vi "proc.util.compare.vi"(8 "error in":errorcluster, 9 "stepElement in":variant, 10 "Input":dbl, 11 "procElement in":variant) -> (0 "error out":errorcluster, 1 "stepElement out":variant, 2 "resulting string":string, 3 "procElement out":variant, 4 "Next State":cluster{"CMD":T1, "data":variant})   [LabVIEW 2024]
uses:
  controls/typeCmdPostStepFunc.ctl
  controls/typeStepVarients.ctl
  Polymorphics/variantCtrlString.vi
  proc.util.validateParamExist.vi
  <vilib>/Utility/error.llb/Clear Errors.vi
  util.error.create.vi
  controls/typeProcVarientName.ctl
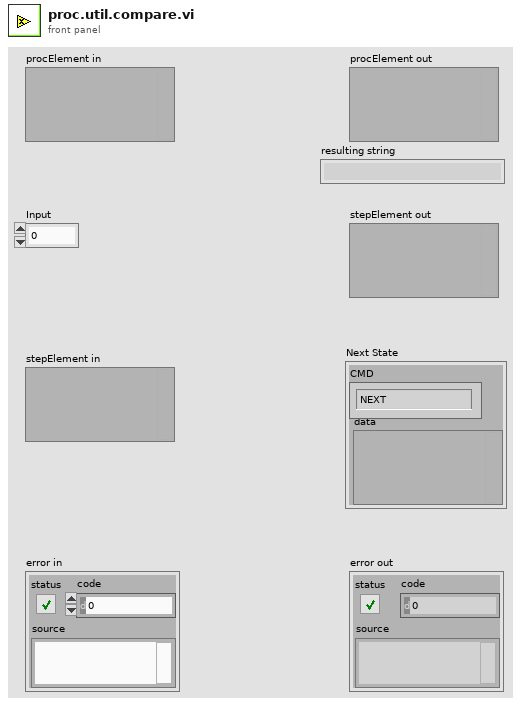
[diagram p1: front panel]
types:
  T1 = typedef "typeCmdPostStepFunc.ctl" = enum16{"NEXT", "PREV", "JUMP", "STAY", "COMPLETE", "ENGCALL.PROC.START", "ENGCALL.PROC.STOP", "ENGCALL.PROC.COMPLETION-CHECK", "ENGCALL.PROC.INIT", "ERROR"}
  T2 = typedef "typeStepVarients.ctl" = enum16{"stepNameID", "stepFunction", "stepReport", "stepSetpoint", "stepPointer", "stepProcPointer", "stepIoPointer", "stepIoValue", "stepFilePointer", "stepMessage", "stepTimeString", "stepNumReg", "stepStrReg", "stepSeconds", "stepUnitDoseParams", "stepUnitIndex"}
  T3 = typedef "typeProcVarientName.ctl" = enum16{"procNameID", "procModuleID", "procPath", "procIsRunning", "procIndex", "procModule", "procRegisterNumeric", "procRegisterString", "procReport", "procReportPrev", "procCLK", "procStepPointer", "procType"}
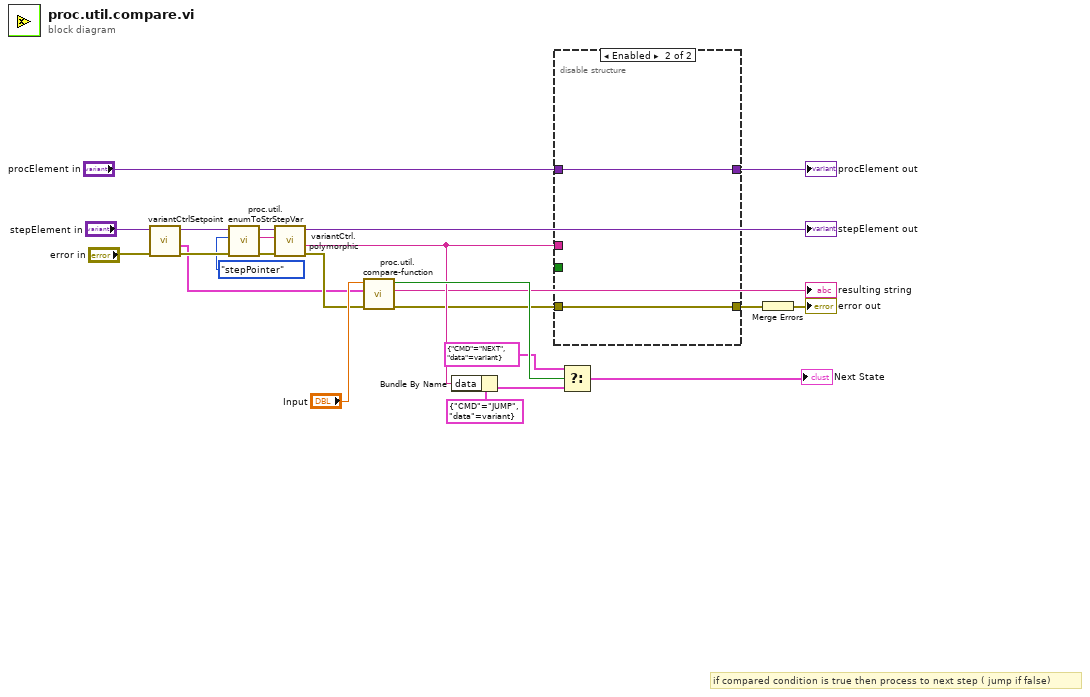
[diagram p0: block diagram]
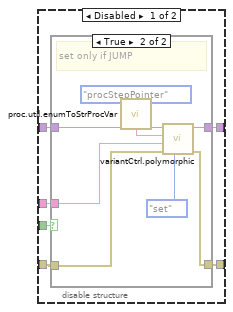
[diagram p2: hidden frame]
diagram:
  # "if compared condition is true then process to next step ( jump if false)"
  n1 = call "variantCtrlSetpoint.vi"("error in"="error in", "procElement in in"="stepElement in") -> ("error out"=w14:errorcluster, "setpoint"=w1:cluster{"Comparison":string, "Setpoint":dbl}, "procElement out"=w15:variant)  [unwired: 6 in, 1 out]
  n2 = call "proc.util.enumToStrStepVar.vi"("Step var"=typeStepVarients."stepPointer") -> ("String"=w12:string)  [unwired: 10 in]
  n3 = call-poly "variantCtrl.polymorphic.vi"("error in"=w14, "name in"=w12, "Step in"=w15) -> ("error out"=w2:errorcluster, "String Value"=w10:string, "Step out"=→"stepElement out":variant)  [unwired: 5 in, 1 out]
  n4 = call "proc.util.compare-function.vi"("error in (no error)"=w2, "input cluster"=w1, "Input"="Input") -> ("error out"=w3:errorcluster, "String"=→"resulting string":string, "Result Condition"=w20:bool)  [unwired: 6 in]
  n5 = Bundle By Name(cluster=cluster{"CMD":T1, "data":variant} {"CMD"=enum."JUMP", "data"=variant} ("JUMP"), "data"=w10) -> (w9:cluster{"CMD":T1, "data":variant})
  n6 = disable-structure shown="Enabled" {
    disable-tunnel: _ -> [w28 _]
    disable-tunnel: "procElement in" -> [w27 w40]
    disable-tunnel: [w26 w40] -> w18
    disable-tunnel: [w25 w39] -> w17
    disable-tunnel: w3 -> [w24 w39]
    disable-tunnel: w10 -> [w23 _]
    frame Disabled {
      n7 = case shown="True" w28 {
        tunnel: w24 -> [w30 w38]
        tunnel: [w30 w35] -> w25
        tunnel: w27 -> [w29 w37]
        tunnel: [w29 w36] -> w26
        tunnel: w23 -> [_ w34]
        frame False {
        }
        frame True {
          # "set only if JUMP"
          n8 = call "proc.util.enumToStrProcVar.vi"("Proc var"=typeProcVarientName."procStepPointer") -> ("String"=w32:string)  [unwired: 10 in]
          n9 = call-poly "variantCtrl.polymorphic.vi"("menu in (get)"=enum16{"get", "set"}."set", "error in"=w38, "String Value"=w34, "name in"=w32, "Step in"=w37) -> ("error out"=w35:errorcluster, "Step out"=w36:variant)  [unwired: 3 in, 2 out]
        }
      }
    }
    frame Enabled {
    }
  }
  "procElement out" <- w18
  n10 = Select(t=cluster{"CMD":T1, "data":variant} {"CMD"=enum."NEXT", "data"=variant} ("NEXT"), s=w20, f=w9) -> (s? t:f=→"Next State":cluster{"CMD":T1, "data":variant})
  n11 = Merge Errors(w17) -> (→"error out":errorcluster)
